vi "Initialise.vi"(8 "error in (no error)":errorcluster, 11 "EventsParent in":refnum<class "Events.lvclass">) -> (0 "error out":errorcluster, 3 "EventsParent out":refnum<class "Events.lvclass">)   [LabVIEW 2020, in "wamplv.lvlib" / "Events.lvclass"]
uses:
  Events.lvclass
  WAMP Client/API/TypeDefs/Connected event data.ctl
  WAMP Client/API/TypeDefs/Disconnected event data.ctl
  WAMP Client/API/TypeDefs/Termination Reason.ctl
  WAMP Client/Private/TypeDef/Termination Reason Enum.ctl
  Events.lvclass/Events.ctl
  WAMP Client/WAMP Client.lvclass
  wamplv.lvlib
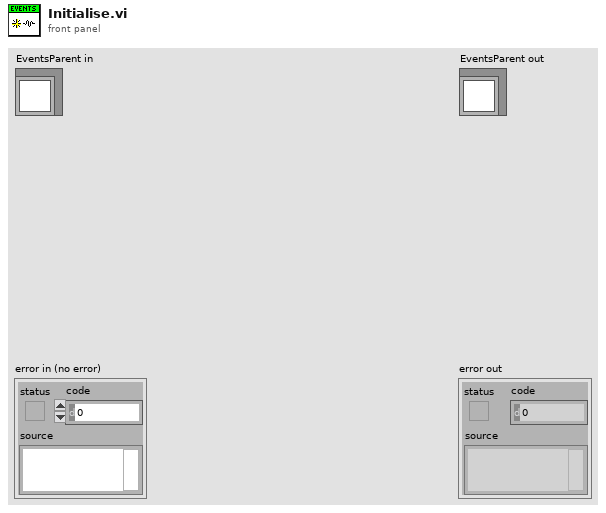
[diagram p1: front panel]
types:
  T1 = typedef "wamplv.lvlib/WAMP Client.lvclass/Connected event data.ctl" = cluster{"Session ID":u64}
  T2 = typedef "wamplv.lvlib/WAMP Client.lvclass/Disconnected event data.ctl" = cluster{"Termination Reason":T3, "Error Out":errorcluster}
  T3 = typedef "wamplv.lvlib/Termination Reason.ctl" = cluster{"Reason":T4, "Reason URI":string, "Message":string}
  T4 = typedef "wamplv.lvlib/WAMP Client.lvclass/Termination Reason Enum.ctl" = enum16{"Goodbye Received", "Abort Received", "Send Goodbye", "Send Abort", "Read Loop Failure", "Write Loop Failure", "Message Loop Failure", "wamplv aborted"}
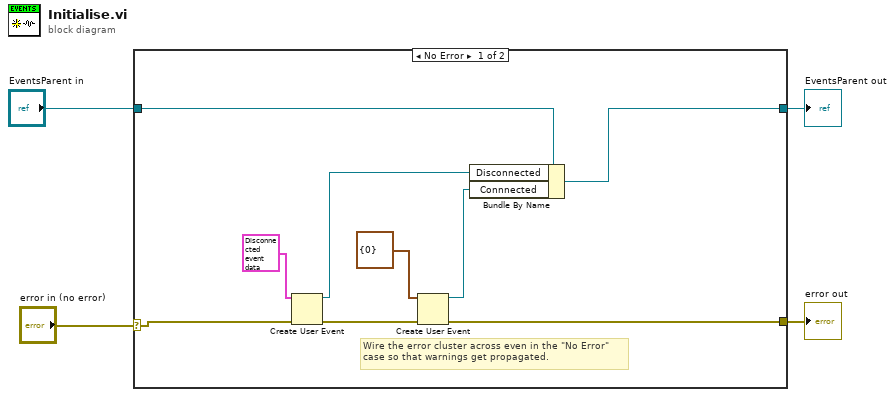
[diagram p0: block diagram]
diagram:
  n1 = case shown="No Error" "error in (no error)" {
    selector: "error in (no error)" -> [w6 w15]
    tunnel: [w5 w15] -> w3
    tunnel: [w12 w14] -> w1
    tunnel: "EventsParent in" -> [w13 w14]
    frame No Error {
      # "Wire the error cluster across even in the \"No Error\"\ncase so that warnings get propagated."
      n2 = Create User Event(user event datatype=T2 {"Termination Reason"={"Reason"=enum."Goodbye Received", "Reason URI"="wamp.error.protocol_violation", "Message"=""}, "Error Out"={"status"=FALSE, "code"=0, "source"=""}} ("Cluster"), error in=w6) -> (user event=w8:refnum<user-event>, error out=w9:errorcluster)
      n3 = Create User Event(user event datatype=T1 {"Session ID"=0} ("Connected event data"), error in=w9) -> (user event=w7:refnum<user-event>, error out=w5:errorcluster)
      n4 = Bundle By Name(cluster=w13, "Disconnected"=w8, "Connnected"=w7) -> (w12:refnum<class "Events.lvclass">)
    }
    frame Error {
    }
  }
  "error out" <- w3
  "EventsParent out" <- w1
